vi "Move.vi"(6 "Direction":T1, 7 "Next Play":u32, 9 "YX Type":string, 11 "Maze 2.0.lvclass":refnum<class "Maze 2.0.lvclass">) -> (1 "Success?":bool)   [LabVIEW 2014, in "Maze 2.0.lvclass"]
uses:
  Maze 2.0.lvclass
  Direction Enum.ctl
  Maze 2.0.lvclass/Maze 2.0.ctl
  Runner Cluster.ctl
  Runner/Runner.lvclass
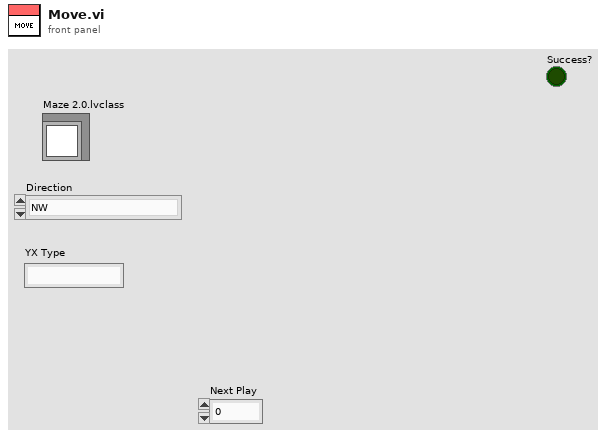
[diagram p1: front panel]
types:
  T1 = typedef "Maze 2.0.lvclass/Direction Enum.ctl" = enum16{"NW", "N", "NE", "E", "SE", "S", "SW", "W"}
  T2 = typedef "Maze 2.0.lvclass/Runner Cluster.ctl" = cluster{"Alive?":bool, "RunnerRef":refnum<data-value>, "TeamIdx":i32, "Player #":i32, "NextPlay":u32}
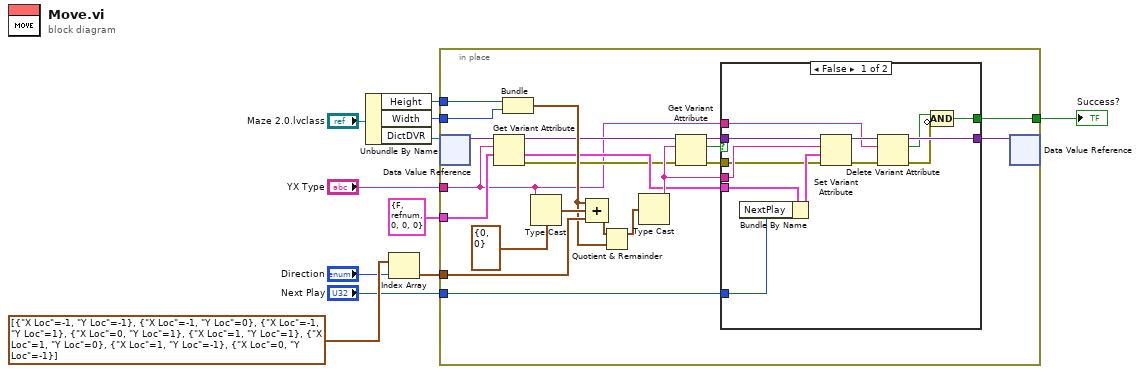
[diagram p0: block diagram]
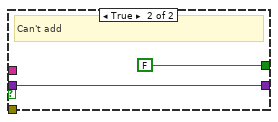
[diagram p2: hidden frame]
diagram:
  n1 = Unbundle By Name("Maze 2.0.lvclass") -> ("Height"=w4:i32, "Width"=w3:i32, "DictDVR"=w5:refnum<data-value>)
  n2 = Index Array(array=cluster{"X Loc":i32, "Y Loc":i32}[] [{"X Loc"=-1, "Y Loc"=-1}, {"X Loc"=-1, "Y Loc"=0}, {"X Loc"=-1, "Y Loc"=1}, {"X Loc"=0, "Y Loc"=1}, {"X Loc"=1, "Y Loc"=1}, {"X Loc"=1, "Y Loc"=0}, {"X Loc"=1, "Y Loc"=-1}, {"X Loc"=0, "Y Loc"=-1}], index="Direction") -> (element=w7:cluster{"X Loc":i32, "Y Loc":i32})
  n3 = in-place {
    in-place-border: "YX Type" -> [w13]
    in-place-border: T2 {"Alive?"=FALSE, "RunnerRef"=refnum, "TeamIdx"=0, "Player #"=0, "NextPlay"=0} ("Cluster") -> [w31]
    in-place-border: w7 -> [w26]
    in-place-border: w4 -> [w30]
    in-place-border: w3 -> [w29]
    in-place-border: [w18] -> w2
    in-place-border: "Next Play" -> [w12]
    n4 = in-place-dvr #1(w5) -> (w32:variant)  [unwired: 1 out]
    n5 = Get Variant Attribute(Variant=w32, name=w13, default value (empty Variant)=w31) -> (duplicate Variant=w22:variant, value=w16:T2, error out=w14:errorcluster)  [unwired: 1 in, 1 out]
    n6 = Bundle("Height"=w30, "Width"=w29) -> (w24:cluster{"Height":i32, "Width":i32})  [unwired: 1 in]
    n7 = Type Cast(type=cluster{"Y":i32, "X":i32} {"Y"=0, "X"=0}, x=w13) -> (*(type *) &x=w25:cluster{"Y":i32, "X":i32})
    n8 = Compound Arithmetic op=ADD(w24, w25, w26) -> (w28:cluster{i32, i32})
    n9 = Quotient & Remainder(x=w28, y=w24) -> (x-y*floor(x/y)=w23:cluster{i32, i32})  [unwired: 1 out]
    n10 = Type Cast(x=w23) -> (*(type *) &x=w17:string)  [unwired: 1 in]
    n11 = Get Variant Attribute(Variant=w22, name=w17, error in=w14) -> (duplicate Variant=w20:variant, found=w21:bool, error out=w15:errorcluster)  [unwired: 1 in, 1 out]
    n12 = case shown="False" w21 {
      tunnel: w20 -> [w45 w47]
      tunnel: [w37 w47] -> w19
      tunnel: [w34 FALSE] -> w18
      tunnel: w17 -> [w44 _]
      tunnel: w16 -> [w43 _]
      tunnel: w15 -> [w41 _]
      tunnel: w13 -> [w38 _]
      tunnel: w12 -> [w33 _]
      frame False {
        n13 = Bundle By Name(cluster=w43, "NextPlay"=w33) -> (w42:T2)
        n14 = Set Variant Attribute(Variant=w45, name=w44, value=w42, error in=w41) -> (Variant out=w40:variant, error out=w39:errorcluster)  [unwired: 1 out]
        n15 = Delete Variant Attribute(4:w39, 6:w38, 7:w40) -> (0:w35:errorcluster, 2:w36:bool, 3:w37:variant)
        n16 = Compound Arithmetic op=AND(w36, invert w35) -> (w34:bool)
      }
      frame True {
        # "Can't add"
      }
    }
    n17 = in-place-dvr #1(w19) -> ()  [unwired: 2 out]
  }
  "Success?" <- w2
